vi "rszvl_core_global.vi"() -> ()   [LabVIEW 2014] (continued)
"Coerce Callback"="", "User Callback"="", "Supported Models"="", "Instrument Options"="", "Repeated Capabilities"="", "Restricted Repeated Capabilities"="", "Help"="This attribute defines the sideband position.\n\nAvailable Repeated Capabilities:\nNone\n\nRemote-control command(s):\n[SENSe<1|2>:]DDEMod:SBANd NORMal | INVerse | AUTO", "Flags"={"OPC Wait"=FALSE, "Dont check status"=FALSE, "*WAI"=FALSE}, "Check Status Callback"=""}, {"Level"=3, "Descriptive Name"="CATV Modulation Standard", "Class Only"=FALSE, "Data Type"=2, "Access"=2, "Identifier"="RSZVL_ATTR_CATV_MODUL_STANDARD", "Range Table"="", "Command"="TV:MST:NAME", "Read Callback"="", "Write Callback"="", "Range Callback"="", "Check Callback"="", "Rngtable Callback"="", "Coerce Callback"="", "User Callback"="", "Supported Models"="", "Instrument Options"="", "Repeated Capabilities"="", "Restricted Repeated Capabilities"="", "Help"="This attribute defines the name for a modulation standard.\n\nAvailable Repeated Capabilities:\nNone\n\nRemote-control command(s):\n[SENSe<1|2>:]TV:MSTandard:NAME", "Flags"={"OPC Wait"=FALSE, "Dont check status"=FALSE, "*WAI"=FALSE}, "Check Status Callback"=""}, {"Level"=3, "Descriptive Name"="CATV Modulation Standard Group Delay", "Class Only"=FALSE, "Data Type"=0, "Access"=2, "Identifier"="RSZVL_ATTR_CATV_MODUL_STANDARD_GDELAY", "Range Table"="rszvl_rngCatvModStandGroupDelay", "Command"="TV:MST:FILT:GDEL", "Read Callback"="", "Write Callback"="", "Range Callback"="", "Check Callback"="", "Rngtable Callback"="", "Coerce Callback"="", "User Callback"="", "Supported Models"="", "Instrument Options"="", "Repeated Capabilities"="", "Restricted Repeated Capabilities"="", "Help"="This attribute defines the group delay for a modulation standard.\n\nAvailable Repeated Capabilities:\nNone\n\nRemote-control command(s):\n[SENSe<1|2>:]TV:MSTandard:FILTer:GDELay", "Flags"={"OPC Wait"=FALSE, "Dont check status"=FALSE, "*WAI"=FALSE}, "Check Status Callback"=""}, {"Level"=3, "Descriptive Name"="CATV Modulation Standard Signal Type", "Class Only"=FALSE, "Data Type"=0, "Access"=2, "Identifier"="RSZVL_ATTR_CATV_MODUL_STANDARD_SIG_TYPE", "Range Table"="rszvl_rngCatvModStandSignalType", "Command"="TV:MST:STYP", "Read Callback"="", "Write Callback"="", "Range Callback"="", "Check Callback"="", "Rngtable Callback"="", "Coerce Callback"="", "User Callback"="", "Supported Models"="", "Instrument Options"="", "Repeated Capabilities"="", "Restricted Repeated Capabilities"="", "Help"="This attribute defines the signal type of a modulation standard.\n\nAvailable Repeated Capabilities:\nNone\n\nRemote-control command(s):\n[SENSe<1|2>:]TV:MSTandard:STYPe", "Flags"={"OPC Wait"=FALSE, "Dont check status"=FALSE, "*WAI"=FALSE}, "Check Status Callback"=""}, {"Level"=2, "Descriptive Name"="ATV Settings", "Class Only"=TRUE, "Data Type"=0, "Access"=0, "Identifier"="", "Range Table"="", "Command"="", "Read Callback"="", "Write Callback"="", "Range Callback"="", "Check Callback"="", "Rngtable Callback"="", "Coerce Callback"="", "User Callback"="", "Supported Models"="", "Instrument Options"="", "Repeated Capabilities"="", "Restricted Repeated Capabilities"="", "Help"="Attributes that configure ATV Settings.\n\n(1) CATV Analog TV Measurement:\nThis attribute defines the analog measurement type.\n\n(2) CATV Analog TV Carrier Measurement:\nThis attribute configures a new carrier or noise measurement with the next sweep for the Carrier–to–Noise Ratio measurement.\n\n(3) CATV Analog TV Carrier Measurement Mode:\nThis attribute defines the measurement method for the Carrier–to–Noise Ratio or Carrier–to–Second Order Beat Ratio measurement.\n\n(4) CATV Analog TV Carrier Bandwidth:\nThis attribute defines the noise reference bandwidth in the C/N measurement.\n\n(5) CATV Analog TV Carrier Next Frequency:\nThis attribute switches from one frequency range to the next according to the measurement frequencies defined by the [SENSe<1|2>:]ATV:CN | CSO | CTB:TABle<1...10>:MFRequencies command.\n\n(6) CATV Analog TV Carrier Noise Floor Correction:\nThis attribute activates or deactivates the noise floor correction.\n\n(7) CATV Analog TV Carrier Reference Channel Manual:\nThis attribute defines the reference channel.\n\n(8) CATV Analog TV Carrier Reference Power Manual:\nThis attribute defines the manual reference power.\n\n(9) CATV Analog TV Carrier Reference Power Mode:\nThis attribute defines the reference power method.\n\n(10) CATV Analog TV Hum Units:\nThis attribute defines the unit of the Hum measurement values.\n\n(11) CATV Analog TV Vision Carrier Power Abs Units:\nThis attribute defines the unit of the absolute vision carrier power.\n\n(12) CATV Analog TV Standard:\nThis attribute sets the TV standard for Analog TV\n\n(13) CATV Analog TV Sound System:\nThis attribute sets the sound system for analog TV measurements.\n\n(14) CATV Analog TV Color:\nThis attribute sets the color system for analog TV measurements.\n\n(15) CATV Analog TV Bar Field:\nThis attribute sets the bar field parameter for analog TV measurements.\n\n(16) CATV Analog TV Bar Line:\nThis attribute sets the bar line parameter for analog TV measurements.\n\n(17) CATV Analog TV Bar Line Type:\nThis attribute sets the bar line type for analog TV measurements.\n\n(18) CATV Analog TV Video Scope Active Field:\nThis attribute defines the active field in the Video Scope measurement.\n\n(19) CATV Analog TV Video Scope Line:\nThis attribute activates triggering at the horizontal sync signal of the indicated line number in the Video Scope measurement..\n\n(20) CATV Analog TV Quiet Line Field:\nThis attribute sets the quiet line field for analog TV measurements.\n\n(21) CATV Analog TV Quiet Line:\nThis attribute sets the quiet line parameter for analog TV measurements.", "Flags"={"OPC Wait"=FALSE, "Dont check status"=FALSE, "*WAI"=FALSE}, "Check Status Callback"=""}, {"Level"=3, "Descriptive Name"="CATV Analog TV Measurement", "Class Only"=FALSE, "Data Type"=0, "Access"=2, "Identifier"="RSZVL_ATTR_CATV_ATV_MEAS", "Range Table"="rszvl_rngCatvAtvMeas", "Command"="CONF:ATV:MEAS", "Read Callback"="", "Write Callback"="", "Range Callback"="", "Check Callback"="", "Rngtable Callback"="", "Coerce Callback"="", "User Callback"="", "Supported Models"="", "Instrument Options"="", "Repeated Capabilities"="", "Restricted Repeated Capabilities"="", "Help"="This attribute defines the analog measurement type.\n\nAvailable Repeated Capabilities:\nNone\n\nRemote-control command(s):\nCONFigure:ATV:MEASurement ASPectrum | CARRiers | CN | CSO | CTB | HUM | VMODulation | VSCope", "Flags"={"OPC Wait"=FALSE, "Dont check status"=FALSE, "*WAI"=FALSE}, "Check Status Callback"=""}, {"Level"=3, "Descriptive Name"="CATV Analog TV Carrier Measurement", "Class Only"=FALSE, "Data Type"=0, "Access"=2, "Identifier"="RSZVL_ATTR_CATV_ATV_CARR_MEAS", "Range Table"="rszvl_rngCatvAtvCarrMeas", "Command"="CONF:ATV:{AtvCarrier}:MEAS", "Read Callback"="", "Write Callback"="", "Range Callback"="", "Check Callback"="", "Rngtable Callback"="", "Coerce Callback"="", "User Callback"="", "Supported Models"="", "Instrument Options"="", "Repeated Capabilities"="", "Restricted Repeated Capabilities"="", "Help"="This attribute configures a new carrier or noise measurement with the next sweep for the Carrier–to–Noise Ratio measurement.\n\nAvailable Repeated Capabilities:\nAtvCarrier: CN,CSO,CTB\r\n\nRemote-control command(s):\nCONFigure:ATV:<CN | CSO | CTB>:MEASurement CARR | NOIS", "Flags"={"OPC Wait"=FALSE, "Dont check status"=FALSE, "*WAI"=FALSE}, "Check Status Callback"=""}, {"Level"=3, "Descriptive Name"="CATV Analog TV Carrier Measurement Mode", "Class Only"=FALSE, "Data Type"=0, "Access"=2, "Identifier"="RSZVL_ATTR_CATV_ATV_MEAS_MODE", "Range Table"="rszvl_rngCatvAtvCarrMeasMode", "Command"="SENS:ATV:{AtvCarrier}:MEAS:MODE", "Read Callback"="", "Write Callback"="", "Range Callback"="", "Check Callback"="", "Rngtable Callback"="", "Coerce Callback"="", "User Callback"="", "Supported Models"="", "Instrument Options"="", "Repeated Capabilities"="", "Restricted Repeated Capabilities"="", "Help"="This attribute defines the measurement method for the Carrier–to–Noise Ratio or Carrier–to–Second Order Beat Ratio measurement.\n\nAvailable Repeated Capabilities:\nAtvCarrier: CN,CSO,CTB\r\n\nRemote-control command(s):\n[SENSe<1|2>:]ATV:<CN | CSO>:MEASurement:MODE ISER | OSER | QLIN", "Flags"={"OPC Wait"=FALSE, "Dont check status"=FALSE, "*WAI"=FALSE}, "Check Status Callback"=""}, {"Level"=3, "Descriptive Name"="CATV Analog TV Carrier Bandwidth", "Class Only"=FALSE, "Data Type"=1, "Access"=2, "Identifier"="RSZVL_ATTR_CATV_ATV_BWID", "Range Table"="rszvl_rngCatvAtvBw", "Command"=":ATV:{AtvCarrier}:BWID", "Read Callback"="", "Write Callback"="", "Range Callback"="", "Check Callback"="", "Rngtable Callback"="", "Coerce Callback"="", "User Callback"="", "Supported Models"="", "Instrument Options"="", "Repeated Capabilities"="", "Restricted Repeated Capabilities"="", "Help"="This attribute defines the noise reference bandwidth in the C/N measurement.\n\nAvailable Repeated Capabilities:\nAtvCarrier: CN,CSO,CTB\r\n\nRemote-control command(s):\n[SENSe<1|2>:]ATV:CN:BWIDth", "Flags"={"OPC Wait"=FALSE, "Dont check status"=FALSE, "*WAI"=FALSE}, "Check Status Callback"=""}, {"Level"=3, "Descriptive Name"="CATV Analog TV Carrier Next Frequency", "Class Only"=FALSE, "Data Type"=4, "Access"=1, "Identifier"="RSZVL_ATTR_CATV_ATV_FREQ_NEXT", "Range Table"="rszvl_rngCatvAtvBw", "Command"=":ATV:{AtvCarrier}:CFR:NEXT", "Read Callback"="", "Write Callback"="", "Range Callback"="", "Check Callback"="", "Rngtable Callback"="", "Coerce Callback"="", "User Callback"="", "Supported Models"="", "Instrument Options"="", "Repeated Capabilities"="", "Restricted Repeated Capabilities"="", "Help"="This attribute switches from one frequency range to the next according to the measurement frequencies defined by the [SENSe<1|2>:]ATV:CN | CSO | CTB:TABle<1...10>:MFRequencies command.\n\nAvailable Repeated Capabilities:\nAtvCarrier: CN,CSO,CTB\r\n\nRemote-control command(s):\n[SENSe<1|2>:]ATV:<CN | CSO | CTB>:CFRelative:NEXT", "Flags"={"OPC Wait"=FALSE, "Dont check status"=FALSE, "*WAI"=FALSE}, "Check Status Callback"=""}, {"Level"=3, "Descriptive Name"="CATV Analog TV Carrier Noise Floor Correction", "Class Only"=FALSE, "Data Type"=3, "Access"=2, "Identifier"="RSZVL_ATTR_CATV_ATV_NOISE_FLOOR_CORRECTION", "Range Table"="", "Command"=":ATV:{AtvCarrier}:POW:NCOR", "Read Callback"="", "Write Callback"="", "Range Callback"="", "Check Callback"="", "Rngtable Callback"="", "Coerce Callback"="", "User Callback"="", "Supported Models"="", "Instrument Options"="", "Repeated Capabilities"="", "Restricted Repeated Capabilities"="", "Help"="This attribute activates or deactivates the noise floor correction.\n\nAvailable Repeated Capabilities:\nAtvCarrier: CN,CSO,CTB\r\n\nRemote-control command(s):\n[SENSe<1|2>:]ATV:<CN | CSO | CTB>:POWer:NCORrection ON | OFF", "Flags"={"OPC Wait"=TRUE, "Dont check status"=FALSE, "*WAI"=FALSE}, "Check Status Callback"=""}, {"Level"=3, "Descriptive Name"="CATV Analog TV Carrier Reference Channel Manual", "Class Only"=FALSE, "Data Type"=0, "Access"=2, "Identifier"="RSZVL_ATTR_CATV_ATV_REF_CHANNEL_MANUAL", "Range Table"="", "Command"=":ATV:{AtvCarrier}:POW:REF:CHAN:MAN", "Read Callback"="", "Write Callback"="", "Range Callback"="", "Check Callback"="", "Rngtable Callback"="", "Coerce Callback"="", "User Callback"="", "Supported Models"="", "Instrument Options"="", "Repeated Capabilities"="", "Restricted Repeated Capabilities"="", "Help"="This attribute defines the reference channel.\n\nAvailable Repeated Capabilities:\nAtvCarrier: CN,CSO,CTB\r\n\nRemote-control command(s):\n[SENSe<1|2>:]ATV:<CN | CSO | CTB>:POWer:REFerence:CHANnel:MANual", "Flags"={"OPC Wait"=FALSE, "Dont check status"=FALSE, "*WAI"=FALSE}, "Check Status Callback"=""}, {"Level"=3, "Descriptive Name"="CATV Analog TV Carrier Reference Power Manual", "Class Only"=FALSE, "Data Type"=1, "Access"=2, "Identifier"="RSZVL_ATTR_CATV_ATV_REF_POWER_MANUAL", "Range Table"="rszvl_rngCatvRelPower", "Command"=":ATV:{AtvCarrier}:POW:REF:MAN", "Read Callback"="", "Write Callback"="", "Range Callback"="", "Check Callback"="", "Rngtable Callback"="", "Coerce Callback"="", "User Callback"="", "Supported Models"="", "Instrument Options"="", "Repeated Capabilities"="", "Restricted Repeated Capabilities"="", "Help"="This attribute defines the manual reference power.\n\nAvailable Repeated Capabilities:\nAtvCarrier: CN,CSO,CTB\r\n\nRemote-control command(s):\n[SENSe<1|2>:]ATV:<CN | CSO | CTB>:POWer:REFerence:MANual", "Flags"={"OPC Wait"=FALSE, "Dont check status"=FALSE, "*WAI"=FALSE}, "Check Status Callback"=""}, {"Level"=3, "Descriptive Name"="CATV Analog TV Carrier Reference Power Mode", "Class Only"=FALSE, "Data Type"=0, "Access"=2, "Identifier"="RSZVL_ATTR_CATV_ATV_REF_POWER_MODE", "Range Table"="rszvl_rngCatvAtvRefPowerMode", "Command"=":ATV:{AtvCarrier}:POW:REF:MODE", "Read Callback"="", "Write Callback"="", "Range Callback"="", "Check Callback"="", "Rngtable Callback"="", "Coerce Callback"="", "User Callback"="", "Supported Models"="", "Instrument Options"="", "Repeated Capabilities"="", "Restricted Repeated Capabilities"="", "Help"="This attribute defines the reference power method.\n\nAvailable Repeated Capabilities:\nAtvCarrier: CN,CSO,CTB\r\n\nRemote-control command(s):\n[SENSe<1|2>:]ATV:<CN | CSO | CTB>:POWer:REFerence:MODE", "Flags"={"OPC Wait"=FALSE, "Dont check status"=FALSE, "*WAI"=FALSE}, "Check Status Callback"=""}, {"Level"=3, "Descriptive Name"="CATV Analog TV Hum Units", "Class Only"=FALSE, "Data Type"=0, "Access"=2, "Identifier"="RSZVL_ATTR_CATV_ATV_HUM_UNIT", "Range Table"="rszvl_rngUnitDbPct", "Command"="CALC:ATV:UNIT:POW:HUM", "Read Callback"="", "Write Callback"="", "Range Callback"="", "Check Callback"="", "Rngtable Callback"="", "Coerce Callback"="", "User Callback"="", "Supported Models"="", "Instrument Options"="", "Repeated Capabilities"="", "Restricted Repeated Capabilities"="", "Help"="This attribute defines the unit of the Hum measurement values.\n\nAvailable Repeated Capabilities:\nNone\n\nRemote-control command(s):\nCALCulate<1|2>:ATV:UNIT:POWer:HUM", "Flags"={"OPC Wait"=FALSE, "Dont check status"=FALSE, "*WAI"=FALSE}, "Check Status Callback"=""}, {"Level"=3, "Descriptive Name"="CATV Analog TV Vision Carrier Power Abs Units", "Class Only"=FALSE, "Data Type"=0, "Access"=2, "Identifier"="RSZVL_ATTR_CATV_ATV_VCP_UNIT", "Range Table"="rszvl_rngCatvPowerUnits", "Command"="CALC:ATV:UNIT:POW:VCP", "Read Callback"="", "Write Callback"="", "Range Callback"="", "Check Callback"="", "Rngtable Callback"="", "Coerce Callback"="", "User Callback"="", "Supported Models"="", "Instrument Options"="", "Repeated Capabilities"="", "Restricted Repeated Capabilities"="", "Help"="This attribute defines the unit of the absolute vision carrier power.\n\nAvailable Repeated Capabilities:\nNone\n\nRemote-control command(s):\nCALCulate<1|2>:ATV:UNIT:POWer:VCPabsolute", "Flags"={"OPC Wait"=FALSE, "Dont check status"=FALSE, "*WAI"=FALSE}, "Check Status Callback"=""}, {"Level"=3, "Descriptive Name"="CATV Analog TV Standard", "Class Only"=FALSE, "Data Type"=0, "Access"=2, "Identifier"="RSZVL_ATTR_CATV_ATV_STANDARD", "Range Table"="rszvl_rngCatvAtvStandard", "Command"="SET:TV:STAN", "Read Callback"="", "Write Callback"="", "Range Callback"="", "Check Callback"="", "Rngtable Callback"="", "Coerce Callback"="", "User Callback"="", "Supported Models"="", "Instrument Options"="", "Repeated Capabilities"="", "Restricted Repeated Capabilities"="", "Help"="This attribute sets the TV standard for Analog TV\n\nAvailable Repeated Capabilities:\nNone\n\nRemote-control command(s):\nSETup:TV:STANdard BG | DK | I | K1 | L | M | N", "Flags"={"OPC Wait"=FALSE, "Dont check status"=FALSE, "*WAI"=FALSE}, "Check Status Callback"=""}, {"Level"=3, "Descriptive Name"="CATV Analog TV Sound System", "Class Only"=FALSE, "Data Type"=0, "Access"=2, "Identifier"="RSZVL_ATTR_CATV_ATV_SOUND_SYSTEM", "Range Table"="rszvl_rngCatvAtvSoundSystem", "Command"="SET:TV:STAN:AUD", "Read Callback"="", "Write Callback"="", "Range Callback"="", "Check Callback"="", "Rngtable Callback"="", "Coerce Callback"="", "User Callback"="", "Supported Models"="", "Instrument Options"="", "Repeated Capabilities"="", "Restricted Repeated Capabilities"="", "Help"="This attribute sets the sound system for analog TV measurements.\n\nAvailable Repeated Capabilities:\nNone\n\nRemote-control command(s):\nSETup:TV:STANdard:AUDio FM55NICAM585 | FM55FM5742 | FM55MONO | FM65NICAM585 | FM65FM6258 | FM65FM6742 | FM65MONO | FM60NICAM6552 | FM60MONO | AM65NICAM585 | AM60MONO | FM45BTSC | FM45EIA_J | FM45FM4742 | FM45MONO", "Flags"={"OPC Wait"=FALSE, "Dont check status"=FALSE, "*WAI"=FALSE}, "Check Status Callback"=""}, {"Level"=3, "Descriptive Name"="CATV Analog TV Color", "Class Only"=FALSE, "Data Type"=0, "Access"=2, "Identifier"="RSZVL_ATTR_CATV_ATV_COLOR", "Range Table"="rszvl_rngCatvAtvColorSystem", "Command"="SET:TV:STAN:COL", "Read Callback"="", "Write Callback"="", "Range Callback"="", "Check Callback"="", "Rngtable Callback"="", "Coerce Callback"="", "User Callback"="", "Supported Models"="", "Instrument Options"="", "Repeated Capabilities"="", "Restricted Repeated Capabilities"="", "Help"="This attribute sets the color system for analog TV measurements.\n\nAvailable Repeated Capabilities:\nNone\n\nRemote-control command(s):\nSETup:TV:STANdard:COLor PAL | NTSC | SECam", "Flags"={"OPC Wait"=FALSE, "Dont check status"=FALSE, "*WAI"=FALSE}, "Check Status Callback"=""}, {"Level"=3, "Descriptive Name"="CATV Analog TV Bar Field", "Class Only"=FALSE, "Data Type"=0, "Access"=2, "Identifier"="RSZVL_ATTR_CATV_ATV_TRIGGER_BAR_FIELD", "Range Table"="rszvl_rngCatvAtvTriggField", "Command"="TRIG{Window}:VID:BFI", "Read Callback"="", "Write Callback"="", "Range Callback"="", "Check Callback"="", "Rngtable Callback"="", "Coerce Callback"="", "User Callback"="", "Supported Models"="", "Instrument Options"="", "Repeated Capabilities"="", "Restricted Repeated Capabilities"="", "Help"="This attribute sets the bar field parameter for analog TV measurements.\n\nAvailable Repeated Capabilities:\nWindow: Win1,Win2\r\n\nRemote-control command(s):\nTRIGger<1|2>[:SEQuence]:VIDeo:BFIeld[:NUMBer]", "Flags"={"OPC Wait"=FALSE, "Dont check status"=FALSE, "*WAI"=FALSE}, "Check Status Callback"=""}, {"Level"=3, "Descriptive Name"="CATV Analog TV Bar Line", "Class Only"=FALSE, "Data Type"=0, "Access"=2, "Identifier"="RSZVL_ATTR_CATV_ATV_TRIGGER_BAR_LINE", "Range Table"="", "Command"="TRIG{Window}:VID:BLIN", "Read Callback"="", "Write Callback"="", "Range Callback"="", "Check Callback"="", "Rngtable Callback"="", "Coerce Callback"="", "User Callback"="", "Supported Models"="", "Instrument Options"="", "Repeated Capabilities"="", "Restricted Repeated Capabilities"="", "Help"="This attribute sets the bar line parameter for analog TV measurements.\n\nAvailable Repeated Capabilities:\nWindow: Win1,Win2\r\n\nRemote-control command(s):\nTRIGger<1|2>[:SEQuence]:VIDeo:BLINe[:NUMBer]", "Flags"={"OPC Wait"=FALSE, "Dont check status"=FALSE, "*WAI"=FALSE}, "Check Status Callback"=""}, {"Level"=3, "Descriptive Name"="CATV Analog TV Bar Line Type", "Class Only"=FALSE, "Data Type"=0, "Access"=2, "Identifier"="RSZVL_ATTR_CATV_ATV_TRIGGER_BAR_LINE_TYPE", "Range Table"="rszvl_rngCatvAtvTriggBarLineType", "Command"="TRIG{Window}:VID:BLIN:TYPE", "Read Callback"="", "Write Callback"="", "Range Callback"="", "Check Callback"="", "Rngtable Callback"="", "Coerce Callback"="", "User Callback"="", "Supported Models"="", "Instrument Options"="", "Repeated Capabilities"="", "Restricted Repeated Capabilities"="", "Help"="This attribute sets the bar line type for analog TV measurements.\n\nAvailable Repeated Capabilities:\nWindow: Win1,Win2\r\n\nRemote-control command(s):\nTRIGger<1|2>[:SEQuence]:VIDeo:BLINe:TYPE", "Flags"={"OPC Wait"=FALSE, "Dont check status"=FALSE, "*WAI"=FALSE}, "Check Status Callback"=""}, {"Level"=3, "Descriptive Name"="CATV Analog TV Video Scope Active Field", "Class Only"=FALSE, "Data Type"=0, "Access"=2, "Identifier"="RSZVL_ATTR_CATV_ATV_TRIGGER_VIDEO_SCOPE_FIELD", "Range Table"="rszvl_rngCatvAtvTriggField", "Command"="TRIG{Window}:VID:FIEL", "Read Callback"="", "Write Callback"="", "Range Callback"="", "Check Callback"="", "Rngtable Callback"="", "Coerce Callback"="", "User Callback"="", "Supported Models"="", "Instrument Options"="", "Repeated Capabilities"="", "Restricted Repeated Capabilities"="", "Help"="This attribute defines the active field in the Video Scope measurement.\n\nAvailable Repeated Capabilities:\nWindow: Win1,Win2\r\n\nRemote-control command(s):\nTRIGger<1|2>[:SEQuence]:VIDeo:FIELd:[NUMBer]", "Flags"={"OPC Wait"=FALSE, "Dont check status"=FALSE, "*WAI"=FALSE}, "Check Status Callback"=""}, {"Level"=3, "Descriptive Name"="CATV Analog TV Video Scope Line", "Class Only"=FALSE, "Data Type"=0, "Access"=2, "Identifier"="RSZVL_ATTR_CATV_ATV_TRIGGER_VIDEO_SCOPE_LINE", "Range Table"="", "Command"="TRIG{Window}:VID:LINE", "Read Callback"="", "Write Callback"="", "Range Callback"="", "Check Callback"="", "Rngtable Callback"="", "Coerce Callback"="", "User Callback"="", "Supported Models"="", "Instrument Options"="", "Repeated Capabilities"="", "Restricted Repeated Capabilities"="", "Help"="This attribute activates triggering at the horizontal sync signal of the indicated line number in the Video Scope measurement..\n\nAvailable Repeated Capabilities:\nWindow: Win1,Win2\r\n\nRemote-control command(s):\nTRIGger<1|2>[:SEQuence]:VIDeo:LINE[:NUMBer]", "Flags"={"OPC Wait"=FALSE, "Dont check status"=FALSE, "*WAI"=FALSE}, "Check Status Callback"=""}, {"Level"=3, "Descriptive Name"="CATV Analog TV Quiet Line Field", "Class Only"=FALSE, "Data Type"=0, "Access"=2, "Identifier"="RSZVL_ATTR_CATV_ATV_TRIGGER_QLINE_FIELD", "Range Table"="rszvl_rngCatvAtvTriggField", "Command"="TRIG{Window}:VID:QFI", "Read Callback"="", "Write Callback"="", "Range Callback"="", "Check Callback"="", "Rngtable Callback"="", "Coerce Callback"="", "User Callback"="", "Supported Models"="", "Instrument Options"="", "Repeated Capabilities"="", "Restricted Repeated Capabilities"="", "Help"="This attribute sets the quiet line field for analog TV measurements.\n\nAvailable Repeated Capabilities:\nWindow: Win1,Win2\r\n\nRemote-control command(s):\nTRIGger<1|2>[:SEQuence]:VIDeo:QFIeld[:NUMBer]", "Flags"={"OPC Wait"=FALSE, "Dont check status"=FALSE, "*WAI"=FALSE}, "Check Status Callback"=""}, {"Level"=3, "Descriptive Name"="CATV Analog TV Quiet Line", "Class Only"=FALSE, "Data Type"=0, "Access"=2, "Identifier"="RSZVL_ATTR_CATV_ATV_TRIGGER_QUIET_LINE", "Range Table"="", "Command"="TRIG{Window}:VID:QLIN", "Read Callback"="", "Write Callback"="", "Range Callback"="", "Check Callback"="", "Rngtable Callback"="", "Coerce Callback"="", "User Callback"="", "Supported Models"="", "Instrument Options"="", "Repeated Capabilities"="", "Restricted Repeated Capabilities"="", "Help"="This attribute sets the quiet line parameter for analog TV measurements.\n\nAvailable Repeated Capabilities:\nWindow: Win1,Win2\r\n\nRemote-control command(s):\nTRIGger<1|2>[:SEQuence]:VIDeo:QLINe[:NUMBer]", "Flags"={"OPC Wait"=FALSE, "Dont check status"=FALSE, "*WAI"=FALSE}, "Check Status Callback"=""}, {"Level"=2, "Descriptive Name"="ATV Limit Settings", "Class Only"=TRUE, "Data Type"=0, "Access"=0, "Identifier"="", "Range Table"="", "Command"="", "Read Callback"="", "Write Callback"="", "Range Callback"="", "Check Callback"="", "Rngtable Callback"="", "Coerce Callback"="", "User Callback"="", "Supported Models"="", "Instrument Options"="", "Repeated Capabilities"="", "Restricted Repeated Capabilities"="", "Help"="Attributes that configure ATV Limit Settings.\n\n(1) CATV Analog TV Frequency Offset Limit:\nThis attribute defines the frequency offset carrier limit.\n\n(2) CATV Analog TV Relative Power Limit:\nThis attribute defines relative power limit\n\n(3) CATV Analog TV Frequency Offset Limit, Vision Carrier :\nThis attribute defines the vision carrier offset limit.\n\n(4) CATV Analog TV Absolute Limit, Vision Carrier:\nThis attribute defines absolute limit of the vision carrier.\n\n(5) CATV Analog TV Carrier to Noise Ratio Limit:\nThis attribute defines the limit for the carrier–to–noise ratio.\n\nNote:\n(1) Only Lower limit is available\n\n(6) CATV Analog TV Carrier to Second Order Beat Ratio Limit:\nThis attribute defines the limit for the carrier–to–second order beat ratio.\n\nNote:\n\n(1) Only Lower Limit is available\n\n(7) CATV Analog TV Carrier to Composite Triple Beat Ratio Lower Limit:\nThis attribute defines the lower limit for the carrier–to–composite triple beat ratio.\n\n(8) CATV Analog TV Hum Limit Lower:\nThis attribute defines the limit for the hum values in dB. If the wrong unit is set, the command produces an execution error. The unit is set via the CALCulate<1|2>:ATV:UNIT:POWer:HUM command.\n\n\n(9) CATV Analog TV Hum Limit Upper:\nThis attribute defines the limit for the hum values in dB. If the wrong unit is set, the command produces an execution error. The unit is set via the CALCulate<1|2>:ATV:UNIT:POWer:HUM command.\n\n(10) CATV Analog TV Modulation Depth Limit, Vision Modulation:\nThis attribute defines the modulation depth limit for the vision modulation.\n\n(11) CATV Analog TV Residual Pictures Limit, Vision Modulation:\nThis attribute defines the limit for the residual picture in the Vision Modulation measurement.\n\n(12) CATV Analog TV Vision Carrier Power Limit, Vision Modulation:\nThis attribute defines the vision carrier power limit in the Vision Modulation measurement.", "Flags"={"OPC Wait"=FALSE, "Dont check status"=FALSE, "*WAI"=FALSE}, "Check Status Callback"=""}, {"Level"=3, "Descriptive Name"="CATV Analog TV Frequency Offset Limit", "Class Only"=FALSE, "Data Type"=1, "Access"=2, "Identifier"="RSZVL_ATTR_CATV_ATV_CARR_LIM_FREQ_OFFSET", "Range Table"="rszvl_rngCatvFreqOffset", "Command"="CALC:ATV:LIM:CARR:{AtvSoundCarrier}IF:{ModifLowUpp}", "Read Callback"="", "Write Callback"="", "Range Callback"="", "Check Callback"="", "Rngtable Callback"="", "Coerce Callback"="", "User Callback"="", "Supported Models"="", "Instrument Options"="", "Repeated Capabilities"="", "Restricted Repeated Capabilities"="", "Help"="This attribute defines the frequency offset carrier limit.\n\nAvailable Repeated Capabilities:\nAtvSoundCarrier: SC1,SC2\r\nModifLowUpp: Low,Upp\r\n\nRemote-control command(s):\nCALCulate<1|2>:ATV:LIMit:CARRiers:<S1IFoffset|S2IFoffset>:<LOWer | UPPer>", "Flags"={"OPC Wait"=FALSE, "Dont check status"=FALSE, "*WAI"=FALSE}, "Check Status Callback"=""}, {"Level"=3, "Descriptive Name"="CATV Analog TV Relative Power Limit", "Class Only"=FALSE, "Data Type"=1, "Access"=2, "Identifier"="RSZVL_ATTR_CATV_ATV_CARR_LIM_REL_POWER", "Range Table"="rszvl_rngCatvRelPower", "Command"="CALC:ATV:LIM:CARR:{AtvSoundCarrier}PR:{ModifLowUpp}", "Read Callback"="", "Write Callback"="", "Range Callback"="", "Check Callback"="", "Rngtable Callback"="", "Coerce Callback"="", "User Callback"="", "Supported Models"="", "Instrument Options"="", "Repeated Capabilities"="", "Restricted Repeated Capabilities"="", "Help"="This attribute defines relative power limit\n\nAvailable Repeated Capabilities:\nAtvSoundCarrier: SC1,SC2\r\nModifLowUpp: Low,Upp\r\n\nRemote-control command(s):\nCALCulate<1|2>:ATV:LIMit:CARRiers:<S1PRelative | S2PRelative>:<LOWer | UPPer>", "Flags"={"OPC Wait"=FALSE, "Dont check status"=FALSE, "*WAI"=FALSE}, "Check Status Callback"=""}, {"Level"=3, "Descriptive Name"="CATV Analog TV Frequency Offset Limit, Vision Carrier", "Class Only"=FALSE, "Data Type"=1, "Access"=2, "Identifier"="RSZVL_ATTR_CATV_ATV_CARR_LIM_VCF", "Range Table"="rszvl_rngCatvFreqOffset", "Command"="CALC:ATV:LIM:CARR:VCF:{ModifLowUpp}", "Read Callback"="", "Write Callback"="", "Range Callback"="", "Check Callback"="", "Rngtable Callback"="", "Coerce Callback"="", "User Callback"="", "Supported Models"="", "Instrument Options"="", "Repeated Capabilities"="", "Restricted Repeated Capabilities"="", "Help"="This attribute defines the vision carrier offset limit.\n\nAvailable Repeated Capabilities:\nModifLowUpp: Low,Upp\r\n\nRemote-control command(s):\nCALCulate<1|2>:ATV:LIMit:CARRiers:VCFoffset:<LOWer | UPPer>", "Flags"={"OPC Wait"=FALSE, "Dont check status"=FALSE, "*WAI"=FALSE}, "Check Status Callback"=""}, {"Level"=3, "Descriptive Name"="CATV Analog TV Absolute Limit, Vision Carrier", "Class Only"=FALSE, "Data Type"=1, "Access"=2, "Identifier"="RSZVL_ATTR_CATV_ATV_CARR_LIM_VCP", "Range Table"="rszvl_rngCatvAbsPower", "Command"="CALC:ATV:LIM:CARR:VCP:{ModifLowUpp}", "Read Callback"="", "Write Callback"="", "Range Callback"="", "Check Callback"="", "Rngtable Callback"="", "Coerce Callback"="", "User Callback"="", "Supported Models"="", "Instrument Options"="", "Repeated Capabilities"="", "Restricted Repeated Capabilities"="", "Help"="This attribute defines absolute limit of the vision carrier.\n\nAvailable Repeated Capabilities:\nModifLowUpp: Low,Upp\r\n\nRemote-control command(s):\nCALCulate<1|2>:ATV:LIMit:CARRiers:VCPabsolute:<LOWer | UPPER>", "Flags"={"OPC Wait"=FALSE, "Dont check status"=FALSE, "*WAI"=FALSE}, "Check Status Callback"=""}, {"Level"=3, "Descriptive Name"="CATV Analog TV Carrier to Noise Ratio Limit", "Class Only"=FALSE, "Data Type"=1, "Access"=2, "Identifier"="RSZVL_ATTR_CATV_ATV_LIM_CN", "Range Table"="rszvl_rngCatvRelPower", "Command"="CALC:ATV:LIM:CN:CN:{ModifLowUpp}", "Read Callback"="", "Write Callback"="", "Range Callback"="", "Check Callback"="", "Rngtable Callback"="", "Coerce Callback"="", "User Callback"="", "Supported Models"="", "Instrument Options"="", "Repeated Capabilities"="", "Restricted Repeated Capabilities"="", "Help"="This attribute defines the limit for the carrier–to–noise ratio.\n\nNote:\n(1) Only Lower limit is available\n\nAvailable Repeated Capabilities:\nModifLowUpp: Low,Upp\r\n\nRemote-control command(s):\nCALCulate<1|2>:ATV:LIMit:CN:CN[:LOWer]", "Flags"={"OPC Wait"=FALSE, "Dont check status"=FALSE, "*WAI"=FALSE}, "Check Status Callback"=""}, {"Level"=3, "Descriptive Name"="CATV Analog TV Carrier to Second Order Beat Ratio Limit", "Class Only"=FALSE, "Data Type"=1, "Access"=2, "Identifier"="RSZVL_ATTR_CATV_ATV_LIM_CSO", "Range Table"="rszvl_rngCatvRelPower", "Command"="CALC:ATV:LIM:CSO:CSO:{ModifLowUpp}", "Read Callback"="", "Write Callback"="", "Range Callback"="", "Check Callback"="", "Rngtable Callback"="", "Coerce Callback"="", "User Callback"="", "Supported Models"="", "Instrument Options"="", "Repeated Capabilities"="", "Restricted Repeated Capabilities"="", "Help"="This attribute defines the limit for the carrier–to–second order beat ratio.\n\nNote:\n\n(1) Only Lower Limit is available\n\nAvailable Repeated Capabilities:\nModifLowUpp: Low,Upp\r\n\nRemote-control command(s):\nCALCulate<1|2>:ATV:LIMit:CSO:CSO[:LOWer]", "Flags"={"OPC Wait"=FALSE, "Dont check status"=FALSE, "*WAI"=FALSE}, "Check Status Callback"=""}, {"Level"=3, "Descriptive Name"="CATV Analog TV Carrier to Composite Triple Beat Ratio Lower Limit", "Class Only"=FALSE, "Data Type"=1, "Access"=2, "Identifier"="RSZVL_ATTR_CATV_ATV_LIM_CTB", "Range Table"="rszvl_rngCatvRelPower", "Command"="CALC:ATV:LIM:CTB:CTB", "Read Callback"="", "Write Callback"="", "Range Callback"="", "Check Callback"="", "Rngtable Callback"="", "Coerce Callback"="", "User Callback"="", "Supported Models"="", "Instrument Options"="", "Repeated Capabilities"="", "Restricted Repeated Capabilities"="", "Help"="This attribute defines the lower limit for the carrier–to–composite triple beat ratio.\n\nAvailable Repeated Capabilities:\nNone\n\nRemote-control command(s):\nCALCulate<1|2>:ATV:LIMit:CTB:CTB[:LOWer]", "Flags"={"OPC Wait"=FALSE, "Dont check status"=FALSE, "*WAI"=FALSE}, "Check Status Callback"=""}, {"Level"=3, "Descriptive Name"="CATV Analog TV Hum Limit Lower", "Class Only"=FALSE, "Data Type"=1, "Access"=2, "Identifier"="RSZVL_ATTR_CATV_ATV_LIM_HUM_LOW", "Range Table"="rszvl_rngCatvHumLimitLower", "Command"="CALC:ATV:LIM:HUM:HUM:LOW", "Read Callback"="", "Write Callback"="", "Range Callback"="", "Check Callback"="", "Rngtable Callback"="", "Coerce Callback"="", "User Callback"="", "Supported Models"="", "Instrument Options"="", "Repeated Capabilities"="", "Restricted Repeated Capabilities"="", "Help"="This attribute defines the limit for the hum values in dB. If the wrong unit is set, the command produces an execution error. The unit is set via the CALCulate<1|2>:ATV:UNIT:POWer:HUM command.\n\nAvailable Repeated Capabilities:\nNone\n\nRemote-control command(s):\nCALCulate<1|2>:ATV:LIMit:HUM:HUM:LOWer", "Flags"={"OPC Wait"=FALSE, "Dont check status"=FALSE, "*WAI"=FALSE}, "Check Status Callback"=""}, {"Level"=3, "Descriptive Name"="CATV Analog TV Hum Limit Upper", "Class Only"=FALSE, "Data Type"=1, "Access"=2, "Identifier"="RSZVL_ATTR_CATV_ATV_LIM_HUM_UPP", "Range Table"="rszvl_rngCatvHumLimitUpper", "Command"="CALC:ATV:LIM:HUM:HUM:UPP", "Read Callback"="", "Write Callback"="", "Range Callback"="", "Check Callback"="", "Rngtable Callback"="", "Coerce Callback"="", "User Callback"="", "Supported Models"="", "Instrument Options"="", "Repeated Capabilities"="", "Restricted Repeated Capabilities"="", "Help"="This attribute defines the limit for the hum values in dB. If the wrong unit is set, the command produces an execution error. The unit is set via the CALCulate<1|2>:ATV:UNIT:POWer:HUM command.\n\nAvailable Repeated Capabilities:\nNone\n\nRemote-control command(s):\nCALCulate<1|2>:ATV:LIMit:HUM:HUM:UPPer", "Flags"={"OPC Wait"=FALSE, "Dont check status"=FALSE, "*WAI"=FALSE}, "Check Status Callback"=""}, {"Level"=3, "Descriptive Name"="CATV Analog TV Modulation Depth Limit, Vision Modulation", "Class Only"=FALSE, "Data Type"=1, "Access"=2, "Identifier"="RSZVL_ATTR_CATV_ATV_LIM_VMOD_MDEP", "Range Table"="rszvl_rngPct", "Command"="CALC:ATV:LIM:VMOD:MDEP:{ModifLowUpp}", "Read Callback"="", "Write Callback"="", "Range Callback"="", "Check Callback"="", "Rngtable Callback"="", "Coerce Callback"="", "User Callback"="", "Supported Models"="", "Instrument Options"="", "Repeated Capabilities"="", "Restricted Repeated Capabilities"="", "Help"="This attribute defines the modulation depth limit for the vision modulation.\n\nAvailable Repeated Capabilities:\nModifLowUpp: Low,Upp\r\n\nRemote-control command(s):\nCALCulate<1|2>:ATV:LIMit:VMODulation:MDEPth:<LOWer | UPPer>", "Flags"={"OPC Wait"=FALSE, "Dont check status"=FALSE, "*WAI"=FALSE}, "Check Status Callback"=""}, {"Level"=3, "Descriptive Name"="CATV Analog TV Residual Pictures Limit, Vision Modulation", "Class Only"=FALSE, "Data Type"=1, "Access"=2, "Identifier"="RSZVL_ATTR_CATV_ATV_LIM_VMOD_RPC", "Range Table"="rszvl_rngPct", "Command"="CALC:ATV:LIM:VMOD:RPC:{ModifLowUpp}", "Read Callback"="", "Write Callback"="", "Range Callback"="", "Check Callback"="", "Rngtable Callback"="", "Coerce Callback"="", "User Callback"="", "Supported Models"="", "Instrument Options"="", "Repeated Capabilities"="", "Restricted Repeated Capabilities"="", "Help"="This attribute defines the limit for the residual picture in the Vision Modulation measurement.\n\nAvailable Repeated Capabilities:\nModifLowUpp: Low,Upp\r\n\nRemote-control command(s):\nCALCulate<1|2>:ATV:LIMit:VMODulation:RPC:<LOWer | UPPer>", "Flags"={"OPC Wait"=FALSE, "Dont check status"=FALSE, "*WAI"=FALSE}, "Check Status Callback"=""}, {"Level"=3, "Descriptive Name"="CATV Analog TV Vision Carrier Power Limit, Vision Modulation", "Class Only"=FALSE, "Data Type"=1, "Access"=2, "Identifier"="RSZVL_ATTR_CATV_ATV_LIM_VMOD_VCP", "Range Table"="rszvl_rngCatvAbsPower", "Command"="CALC:ATV:LIM:VMOD:VCP:{ModifLowUpp}", "Read Callback"="", "Write Callback"="", "Range Callback"="", "Check Callback"="", "Rngtable Callback"="", "Coerce Callback"="", "User Callback"="", "Supported Models"="", "Instrument Options"="", "Repeated Capabilities"="", "Restricted Repeated Capabilities"="", "Help"="This attribute defines the vision carrier power limit in the Vision Modulation measurement.\n\nAvailable Repeated Capabilities:\nModifLowUpp: Low,Upp\r\n\nRemote-control command(s):\nCALCulate<1|2>:ATV:LIMit:VMODulation:VCPower:<LOWer | UPPer>", "Flags"={"OPC Wait"=FALSE, "Dont check status"=FALSE, "*WAI"=FALSE}, "Check Status Callback"=""}, {"Level"=2, "Descriptive Name"="ATV Limit Results", "Class Only"=TRUE, "Data Type"=0, "Access"=0, "Identifier"="", "Range Table"="", "Command"="", "Read Callback"="", "Write Callback"="", "Range Callback"="", "Check Callback"="", "Rngtable Callback"="", "Coerce Callback"="", "User Callback"="", "Supported Models"="", "Instrument Options"="", "Repeated Capabilities"="", "Restricted Repeated Capabilities"="", "Help"="Attributes that return ATV limit results.\n\n(1) CATV Analog TV Frequency Offset Limit Result:\nThis attribute performs a limit check for the frequency offset of the sound carrier.\n\n(2) CATV Analog TV Relative Power Limit Result:\nThis attribute performs an limit check for the relative power of the sound carrier.\n\n(3) CATV Analog TV Frequency Offset Limit, Vision Carrier Result:\nThis attribute performs a limit check for the frequency offset of the vision carrier.\n\n(4) CATV Analog TV Absolute Limit, Vision Carrier Result:\nThis attribute performs a limit check for the absolute vision carrier power.\n\n(5) CATV Analog TV Carrier to Noise Ratio Limit Result:\nThis attribute performs a limit check for the carrier–to–noise ratio.\n\nNote:\n\n(1) Only Lower Limit is available.\n\n(6) CATV Analog TV Carrier to Second Order Beat Ratio Limit Result:\nThis attribute performs a limit check for the carrier–to–second order beat ratio.\n\nNote:\n\n(1) Only Lower Limit is available\n\n(7) CATV Analog TV Carrier to Composite Triple Beat Ratio Limit Result:\nThis attribute performs a limit check for the carrier–to–composite triple beat ratio.\n\nNote:\n\n(1) Only Lower Limit is available.\n\n(8) CATV Analog TV Hum Limit Result:\nThis attribute performs a limit check for the Hum measurement.\n\n(9) CATV Analog TV Vision Modulation Result:\nThis attribute performs a limit check for the  Vision Modulation measurement.", "Flags"={"OPC Wait"=FALSE, "Dont check status"=FALSE, "*WAI"=FALSE}, "Check Status Callback"=""}, {"Level"=3, "Descriptive Name"="CATV Analog TV Frequency Offset Limit Result", "Class Only"=FALSE, "Data Type"=0, "Access"=0, "Identifier"="RSZVL_ATTR_CATV_ATV_CARR_LIM_FREQ_OFFSET_RESULT", "Range Table"="rszvl_rngCatvResults", "Command"="CALC:ATV:LIM:RES:CARR:{AtvSoundCarrier}IF:{ModifLowUpp}?", "Read Callback"="", "Write Callback"="", "Range Callback"="", "Check Callback"="", "Rngtable Callback"="", "Coerce Callback"="", "User Callback"="", "Supported Models"="", "Instrument Options"="", "Repeated Capabilities"="", "Restricted Repeated Capabilities"="", "Help"="This attribute performs a limit check for the frequency offset of the sound carrier.\n\nAvailable Repeated Capabilities:\nAtvSoundCarrier: SC1,SC2\r\nModifLowUpp: Low,Upp\r\n\nRemote-control command(s):\nCALCulate<1|2>:ATV:LIMit:RESult:CARRiers:<S1IFoffset | S2IFoffset>:<LOWer | UPPer>?", "Flags"={"OPC Wait"=FALSE, "Dont check status"=FALSE, "*WAI"=FALSE}, "Check Status Callback"=""}, {"Level"=3, "Descriptive Name"="CATV Analog TV Relative Power Limit Result", "Class Only"=FALSE, "Data Type"=0, "Access"=0, "Identifier"="RSZVL_ATTR_CATV_ATV_CARR_LIM_REL_POWER_RESULT", "Range Table"="rszvl_rngCatvResults", "Command"="CALC:ATV:LIM:RES:CARR:{AtvSoundCarrier}PR:{ModifLowUpp}?", "Read Callback"="", "Write Callback"="", "Range Callback"="", "Check Callback"="", "Rngtable Callback"="", "Coerce Callback"="", "User Callback"="", "Supported Models"="", "Instrument Options"="", "Repeated Capabilities"="", "Restricted Repeated Capabilities"="", "Help"="This attribute performs an limit check for the relative power of the sound carrier.\n\nAvailable Repeated Capabilities:\nAtvSoundCarrier: SC1,SC2\r\nModifLowUpp: 
